vi "Open Report file.vi"(8 "error in (no error)":errorcluster, 10 "Report file path":path, 11 "Report In":refnum<class "Test Report.lvclass">) -> (0 "error out":errorcluster, 3 "Report Out":refnum<class "Test Report.lvclass">)   [LabVIEW 2020, in "Test Report.lvclass"]
uses:
  Test Report.lvclass
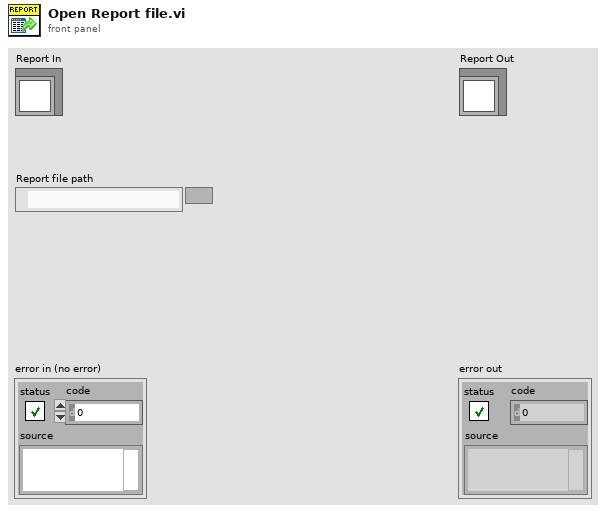
[diagram p1: front panel]
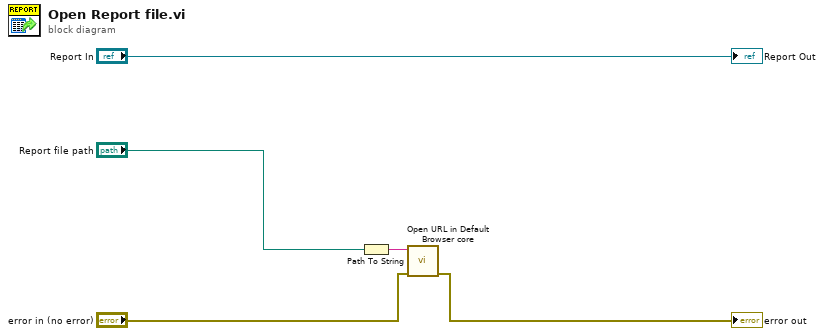
[diagram p0: block diagram]
diagram:
  n1 = Path To String(path="Report file path") -> (string=w1:string)
  n2 = call <vilib>:"Open URL in Default Browser core.vi"("error in (no error)"="error in (no error)", "url"=w1) -> ("error out"=→"error out":errorcluster)  [unwired: 4 in, 1 out]
  "Report Out" <- "Report In"
